vi "Server Connection Loop.vi"(8 "error in (no error)":errorcluster, 11 "TCPMessaging in":refnum<class "TCPMessaging.lvclass">) -> (0 "error out":errorcluster)   [LabVIEW 2020, in "Vecto.lvlib" / "TCPMessaging.lvclass"]
doc: "Listens for new incoming connections and spawns async client loops. The async client loops handle the handshake with the client app."
uses:
  TCPMessaging.lvclass
  TCPMessaging.lvclass/TCPMessaging.ctl
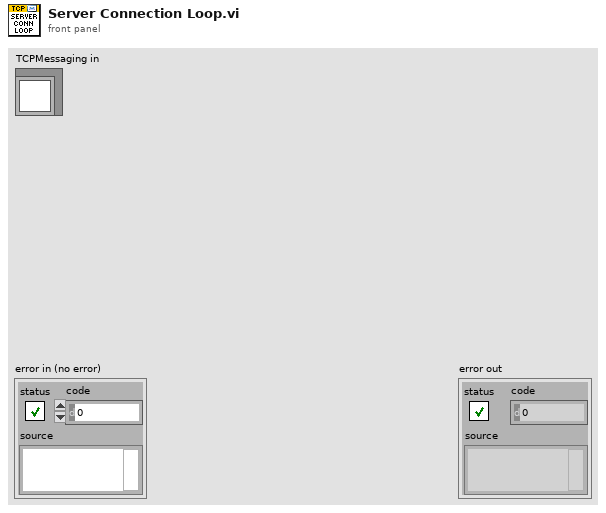
[diagram p1: front panel]
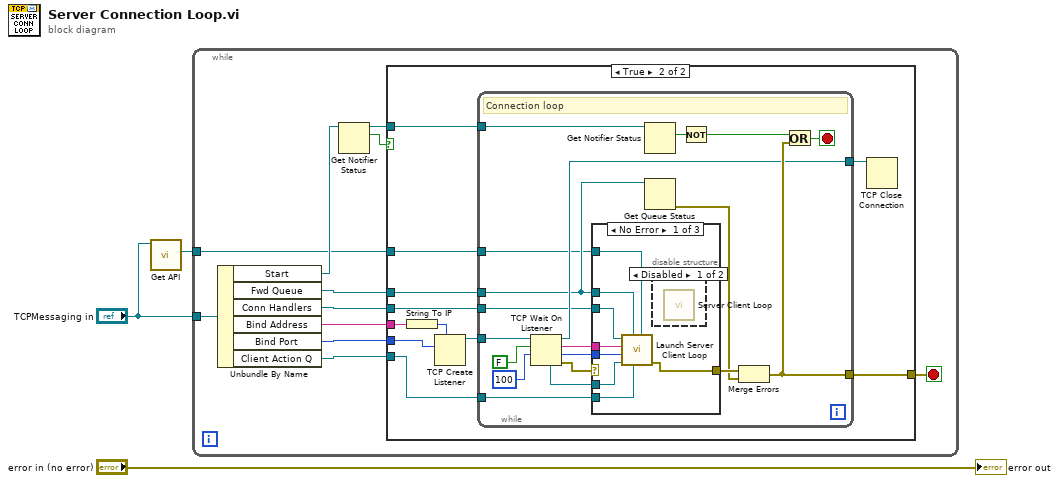
[diagram p0: block diagram]
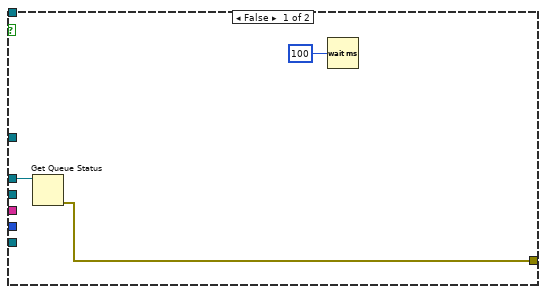
[diagram p2: hidden frame]
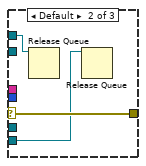
[diagram p4: hidden frame]
diagram:
  n1 = call "Get API.vi"("TCPMessaging in"="TCPMessaging in") -> ("TCP Messaging API"=w1:refnum<class "TCPMessageAPI.lvclass">)  [unwired: 8 in, 2 out]
  n2 = while {
    tunnel: "TCPMessaging in" -> [w11]
    tunnel: w1 -> [w5]
    stop <- w6 stop-if-true
    n3 = Unbundle By Name(w11) -> ("Start"=w9:refnum<notifier>, "Fwd Queue"=w12:refnum<queue>, "Conn Handlers"=w4:refnum<queue>, "Bind Address"=w14:string, "Bind Port"=w13:u16, "Client Action Q"=w10:refnum<queue>)
    n4 = Get Notifier Status(notifier=w9) -> (notifier out=w8:refnum<notifier>, current notification=w7:bool)  [unwired: 1 in, 3 out]
    n5 = case shown="True" w7 {
      tunnel: w14 -> [_ w28]
      tunnel: w13 -> [_ w27]
      tunnel: w12 -> [w16 w24]
      tunnel: w10 -> [_ w23]
      tunnel: w8 -> [_ w22]
      tunnel: [w15 w20] -> w6
      tunnel: w5 -> [_ w19]
      tunnel: w4 -> [_ w18]
      frame False {
        n6 = Get Queue Status(queue=w16) -> (error out=w15:errorcluster)  [unwired: 2 in, 7 out]
        n7 = Wait (ms)(milliseconds to wait=u32 100) -> ()  [unwired: 1 out]
      }
      frame True {
        n8 = String To IP(1:w28) -> (0:w26:u32)
        n9 = TCP Create Listener(7:w26, 10:w27) -> (3:w25:refnum<k5>)  [unwired: 3 in, 2 out]
        n10 = while {
          tunnel: w25 -> [w42]
          tunnel: w24 -> [w31]
          tunnel: w23 -> [w38]
          tunnel: w22 -> [w36]
          tunnel: [w34] -> w21
          tunnel: [w47] -> w20
          tunnel: w19 -> [w30]
          tunnel: w18 -> [w29]
          stop <- w37 stop-if-true
          # "Connection loop"
          n11 = TCP Wait On Listener(9:100 ("timeout ms (wait forever: -1)"), 10:FALSE ("resolve remote address (T)"), 11:w42) -> (0:w43:errorcluster, 1:w41:u16, 2:w40:string, 3:w34:refnum<k5>, 4:w39:refnum<k5>)  [unwired: 1 in]
          n12 = case shown="No Error" w43 {
            selector: w43 -> [_ w58 _]
            tunnel: w41 -> [w54 _ _]
            tunnel: w40 -> [w55 _ _]
            tunnel: w39 -> [w53 _ _]
            tunnel: w31 -> [w51 w56 _]
            tunnel: w38 -> [w52 w57 _]
            tunnel: [w50 w58 _] -> w46
            tunnel: w30 -> [w49 _ _]
            tunnel: w29 -> [w48 _ _]
            frame No Error {
              n13 = call "Launch Server Client Loop.vi"("TCPMessageAPI"=w49, "Client Action Q"=w52, "Fwd Queue"=w51, "TCP Client"=w53, "Remote Port"=w54, "Remote Address"=w55, "Conn Handlers"=w48) -> ("error out"=w50:errorcluster)  [unwired: 4 in]
              n14 = disable-structure shown="Disabled" {
                frame Disabled {
                  n15 = call "Server Client Loop.vi"() -> ()  [unwired: 12 in]
                }
                frame Enabled {
                }
              }
            }
            frame Default {
              n16 = Release Queue(queue=w56) -> ()  [unwired: 2 in, 3 out]
              n17 = Release Queue(queue=w57) -> ()  [unwired: 2 in, 3 out]
            }
            frame Error {
            }
          }
          n18 = Get Notifier Status(notifier=w36) -> (current notification=w35:bool)  [unwired: 1 in, 4 out]
          n19 = Get Queue Status(queue=w31) -> (error out=w32:errorcluster)  [unwired: 2 in, 7 out]
          n20 = Not(x=w35) -> (.not. x?=w33:bool)
          n21 = Merge Errors(w46, w32) -> (w47:errorcluster)
          n22 = Or(x=w33, y=w47) -> (x .or. y?=w37:bool)
        }
        n23 = TCP Close Connection(connection ID=w21) -> ()  [unwired: 2 in, 2 out]
      }
    }
  }
  "error out" <- "error in (no error)"
